vi "create_a_SCAN.vi"() -> ()   [LabVIEW 2013]
uses:
  <vilib>/Analysis/Matrix/Datatypes/RealMatrix.ctl
  <vilib>/Analysis/Matrix/NI_Matrix.lvlib
panel:
  in  "Bouton OK":bool
  in  "Where to save":path=path "D:/par_dates"
  out "stored XY":T1
  out "Graphe XY":T2(graph)
  out "final XY":T1
  in  "Number of Positions":u32=40
  in  "Spacing Y (µm)":dbl=100.0 step=0.001
  in  "Spacing X (µm)":dbl=100.0 step=0.001
  in  "Method":u8(ring) items=["Spiral Scan", "Column Scan", "Line Scan"]
  out "Field\nHeigth (µm)":dbl
  out "Field\nWidth (µm)":dbl
  in  "Microscope Objective\nMagnification":dbl=60.0 min=1.0 max=1000.0 step=1.0
  # "X"
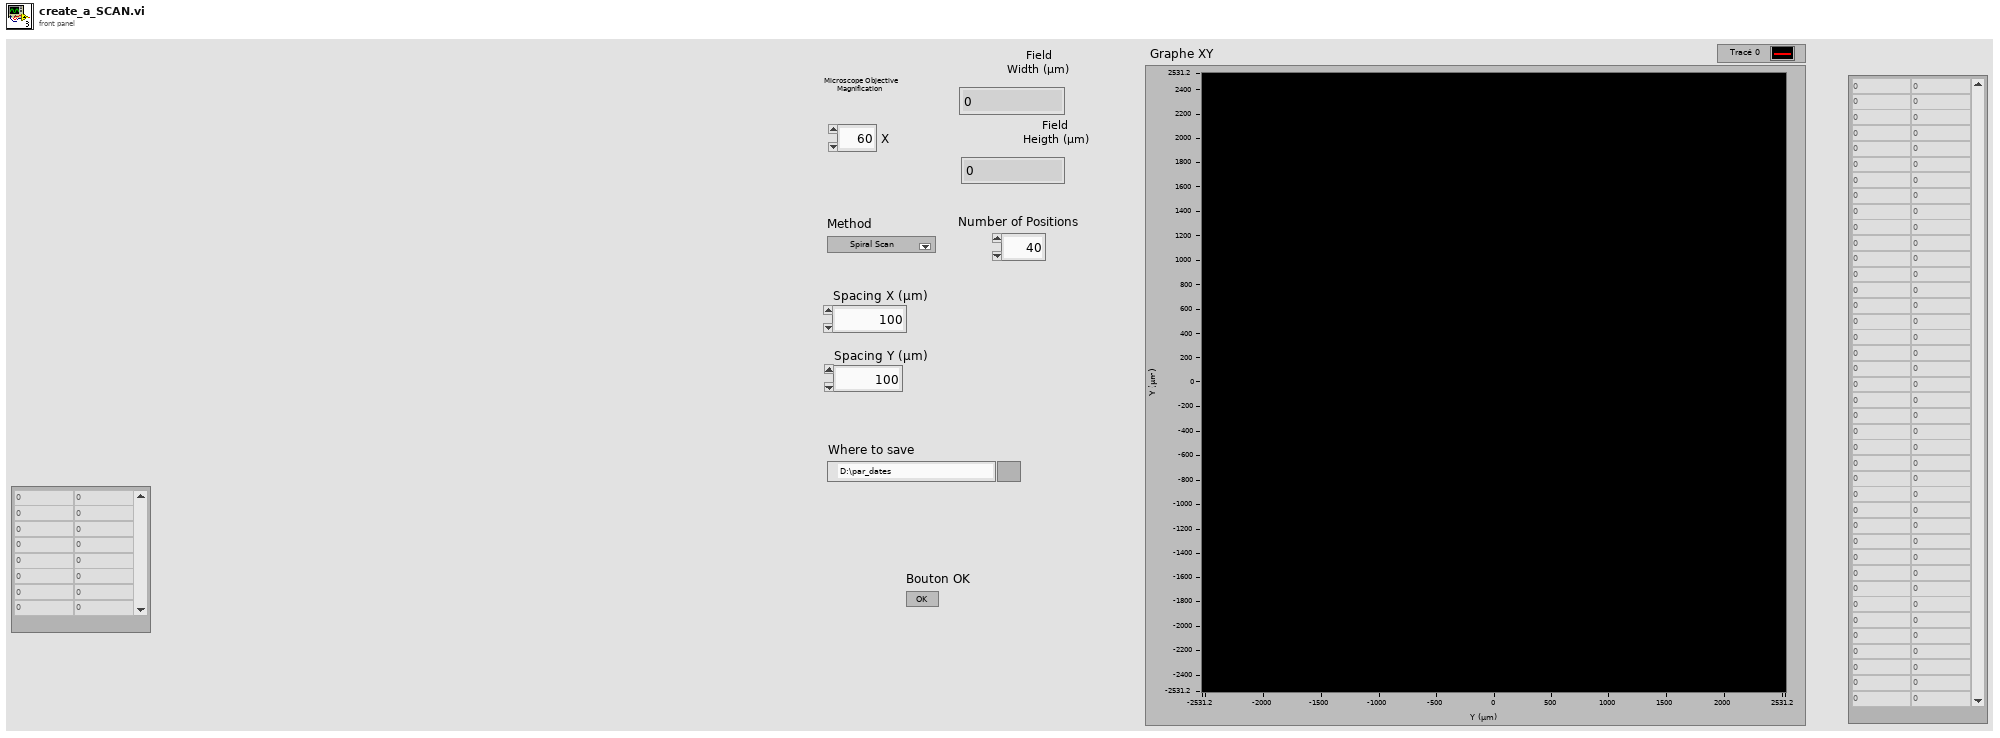
[diagram p1: front panel]
types:
  T1 = typedef "NI_Matrix.lvlib/RealMatrix.ctl" = dbl[][]
  T2 = cluster{cluster{"Real Matrix Element":dbl, "Real Matrix Element":dbl}[]}[]
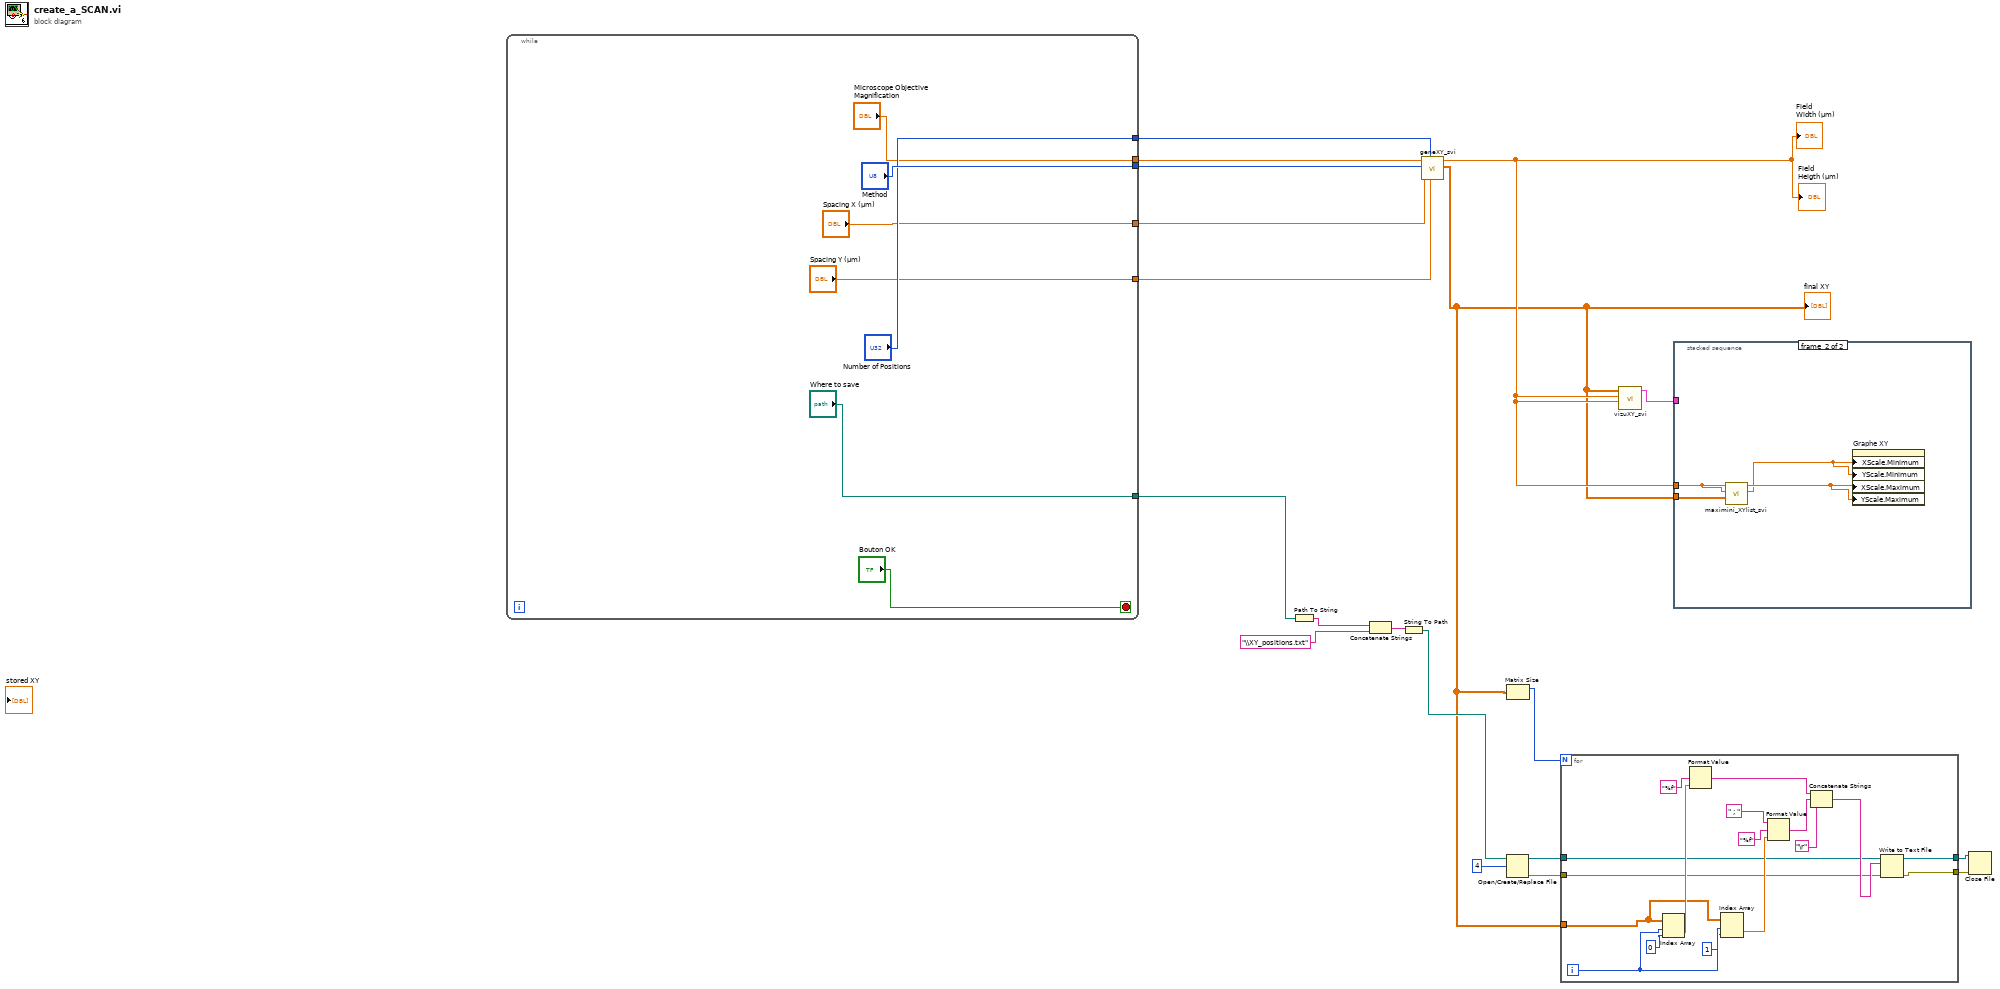
[diagram p0: block diagram]
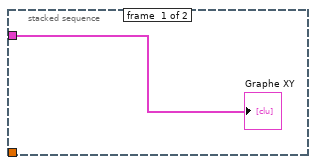
[diagram p2: hidden frame]
diagram:
  n1 = while {
    tunnel: ["Method"] -> w19
    tunnel: ["Number of Positions"] -> w18
    tunnel: ["Spacing Y (µm)"] -> w17
    tunnel: ["Spacing X (µm)"] -> w15
    tunnel: ["Microscope Objective\nMagnification"] -> w14
    tunnel: ["Where to save"] -> w1
    stop <- "Bouton OK" stop-if-true
  }
  n2 = Path To String(path=w1) -> (string=w11:string)
  n3 = Concatenate Strings(w11, "\\XY_positions.txt") -> (w10:string)
  n4 = String To Path(string=w10) -> (path=w4:path)
  n5 = call "geneXY_svi.vi"("Spacing Y (µm)"=w17, "Number of Positions"=w18, "Spacing X (µm)"=w15, "Method"=w19, "Microscope Objective\nMagnification"=w14) -> ("Real Matrix"=w3:T1, "field_size(µm)"=w13:dbl)  [unwired: 5 in]
  "Field\nWidth (µm)" <- w13
  "Field\nHeigth (µm)" <- w13
  "final XY" <- w3
  n6 = Open/Create/Replace File(file path (use dialog)=w4, operation (0:open)=4) -> (refnum out=w8:refnum<file>, error out=w7:errorcluster)  [unwired: 4 in, 1 out]
  n7 = Matrix Size(0:w3) -> (1:w2:i32)  [unwired: 1 out]
  n8 = for {
    N: w2 -> [_]
    tunnel: w8 -> [w32]
    tunnel: w7 -> [w31]
    tunnel: [w30] -> w6
    tunnel: [w29] -> w5
    tunnel: w3 -> [w27]
    i -> [w40]
    n9 = Index Array(array=w27, index (row)=w40, index (col)=0) -> (element=w42:dbl)
    n10 = Format Value(format string="%f" ("chaîne"), value (0)=w42) -> (output string=w35:string)  [unwired: 1 in]
    n11 = Index Array(array=w27, index (row)=w40, index (col)=1) -> (element=w37:dbl)
    n12 = Format Value(string ("")=" ; ", format string="%f" ("chaîne"), value (0)=w37) -> (output string=w34:string)
    n13 = Concatenate Strings(w35, w34, "\r") -> (w33:string)
    n14 = Write to Text File(file (use dialog)=w32, text=w33, error in=w31) -> (refnum out=w30:refnum<file>, error out=w29:errorcluster)  [unwired: 1 in, 1 out]
  }
  n15 = call "vizuXY_svi.vi"("LY (mm)"=w13, "LX (mm)"=w13, "stored XY (µm)"=w3) -> ("Tableau"=w16:T2)  [unwired: 8 in]
  n16 = stacked-sequence {
    tunnel: w16 -> [w44 _]
    tunnel: w13 -> [_ w46]
    tunnel: w3 -> [_ w45]
    frame #0 {
      "Graphe XY" <- w44
    }
    frame #1 {
      n17 = call "maximini_XYlist_svi.vi"("stored XY"=w45, "LY"=w46, "LX"=w46) -> ("mini (µm)"=w47:dbl, "maxi (µm)"=w48:dbl)  [unwired: 7 in]
      n18 = property on="Graphe XY" class="GraphXY (strict)"("XScale.Minimum"=w47, "YScale.Minimum"=w47, "XScale.Maximum"=w48, "YScale.Maximum"=w48) -> ()  [unwired: 2 in, 2 out]
    }
  }
  n19 = Close File(refnum=w6, error in=w5) -> ()  [unwired: 2 out]
